vi "XUVCCDRotate.vi"() -> ()   [LabVIEW 2017]
uses:
  <vilib>/Utility/file.llb/Write Delimited Spreadsheet (DBL).vi
  atmcd32d.dll
panel:
  out "Array":dbl[](array[numeric])
  in  "Nb of steps":i32=50000
  out "Current position":dbl
  in  "Step size (deg.)":dbl=10.0
  out "Is Ready?":bool
  out "VISA resource name":refnum<visa-resource-name>="ASRL7::INSTR"
  out "Connected":bool
  in  "start":bool
  in  "?":bool
  out "Status":u32
  out "Get Status":u32
  out "Vertical Binned Waveform Graph":i32[](graph)
  in  "Numeric":dbl
  out "Intensity Graph":i32[][](graph)
  out "Set Image":u32
  out "Set Gate Mode":u32
  out "Shut Down":u32
  out "Detector Y Pixels":i32
  out "Get Detector":u32
  out "Set Exposure Time":u32
  out "Set Trigger Mode":u32
  out "Set Readout Mode":u32
  out "Set Acquisition Mode":u32
  out "Check Timings":u32
  out "Detector X Pixels":i32
  out "Start Acquisition":u32
  out "Get Acquired Data":u32
  out "Calculated Exposure Value":sgl format="%.5f"
  in  "Exposure Time (secs)":sgl format="%.2f"
  out "Initialize":u32
  in  "Trigger":u32(ring) items=["Internal", "External"]
  # "Status"
  # "Return values"
  # "USB iStarIMAG32at.VI"
  # "Acquisition Mode: Single Scan\nReadout Mode: Full Resolution Image"
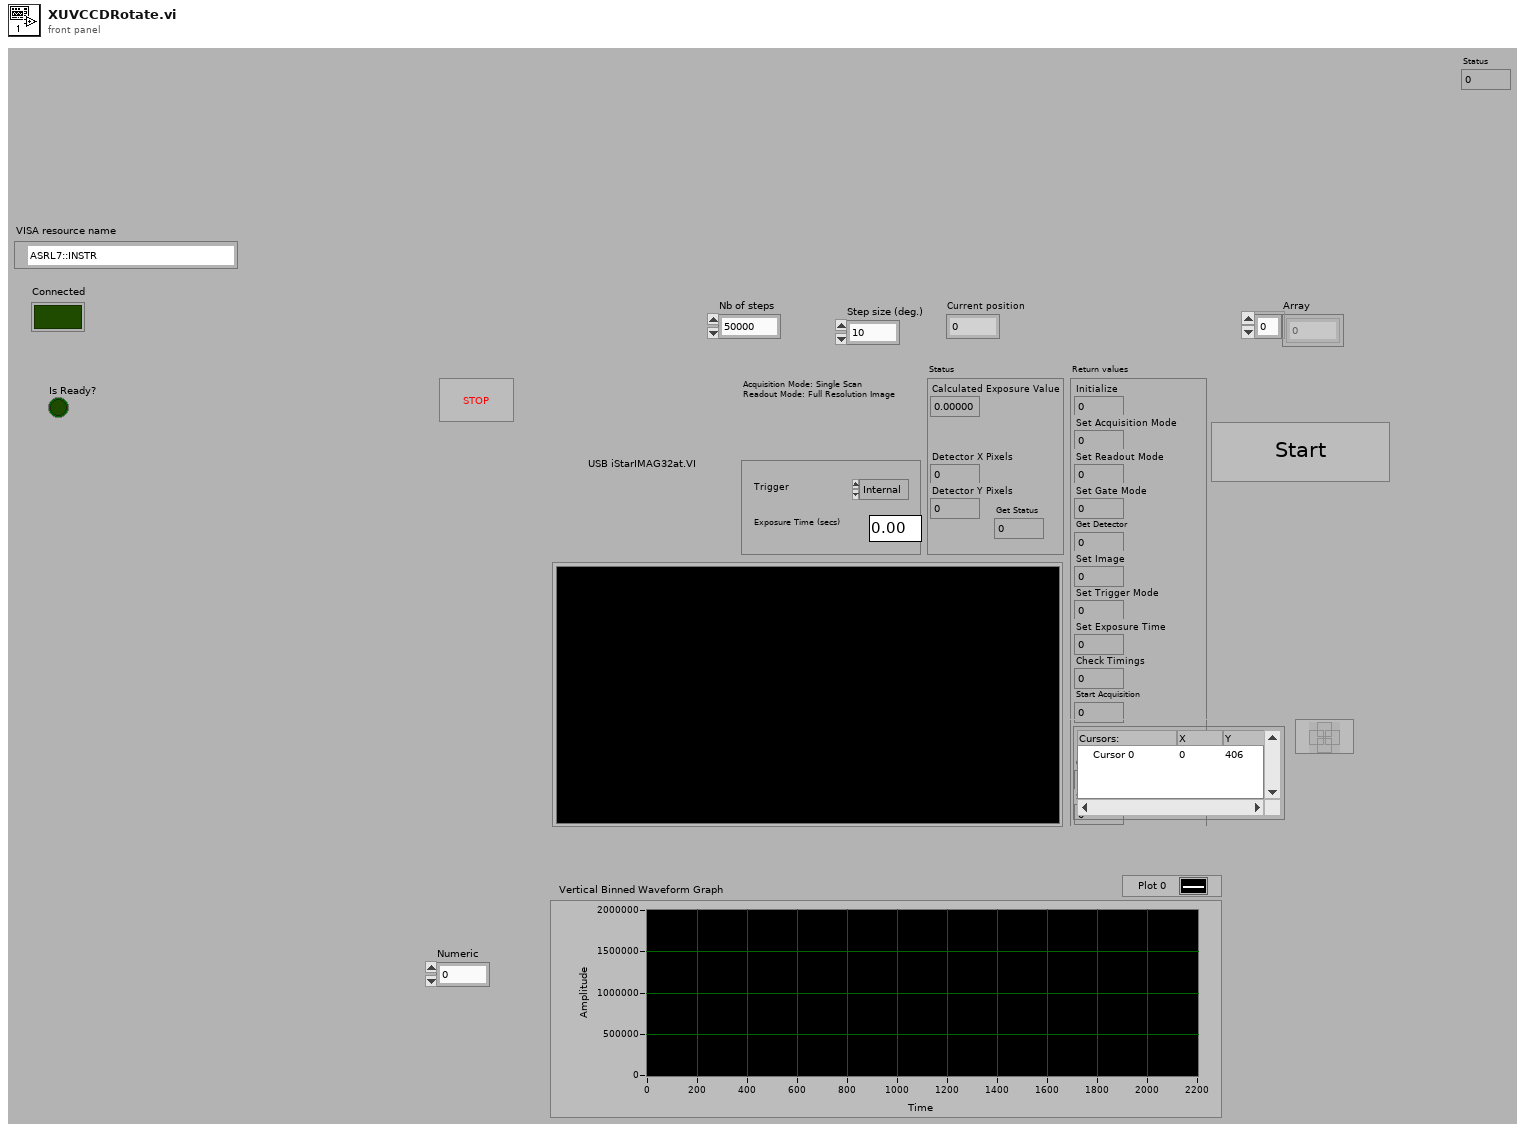
[diagram p1: front panel]
types:
  T1 = cluster{"VISA resource name":refnum<visa-resource-name>, "Device name":string, "Controller address":i32, "error":errorcluster}
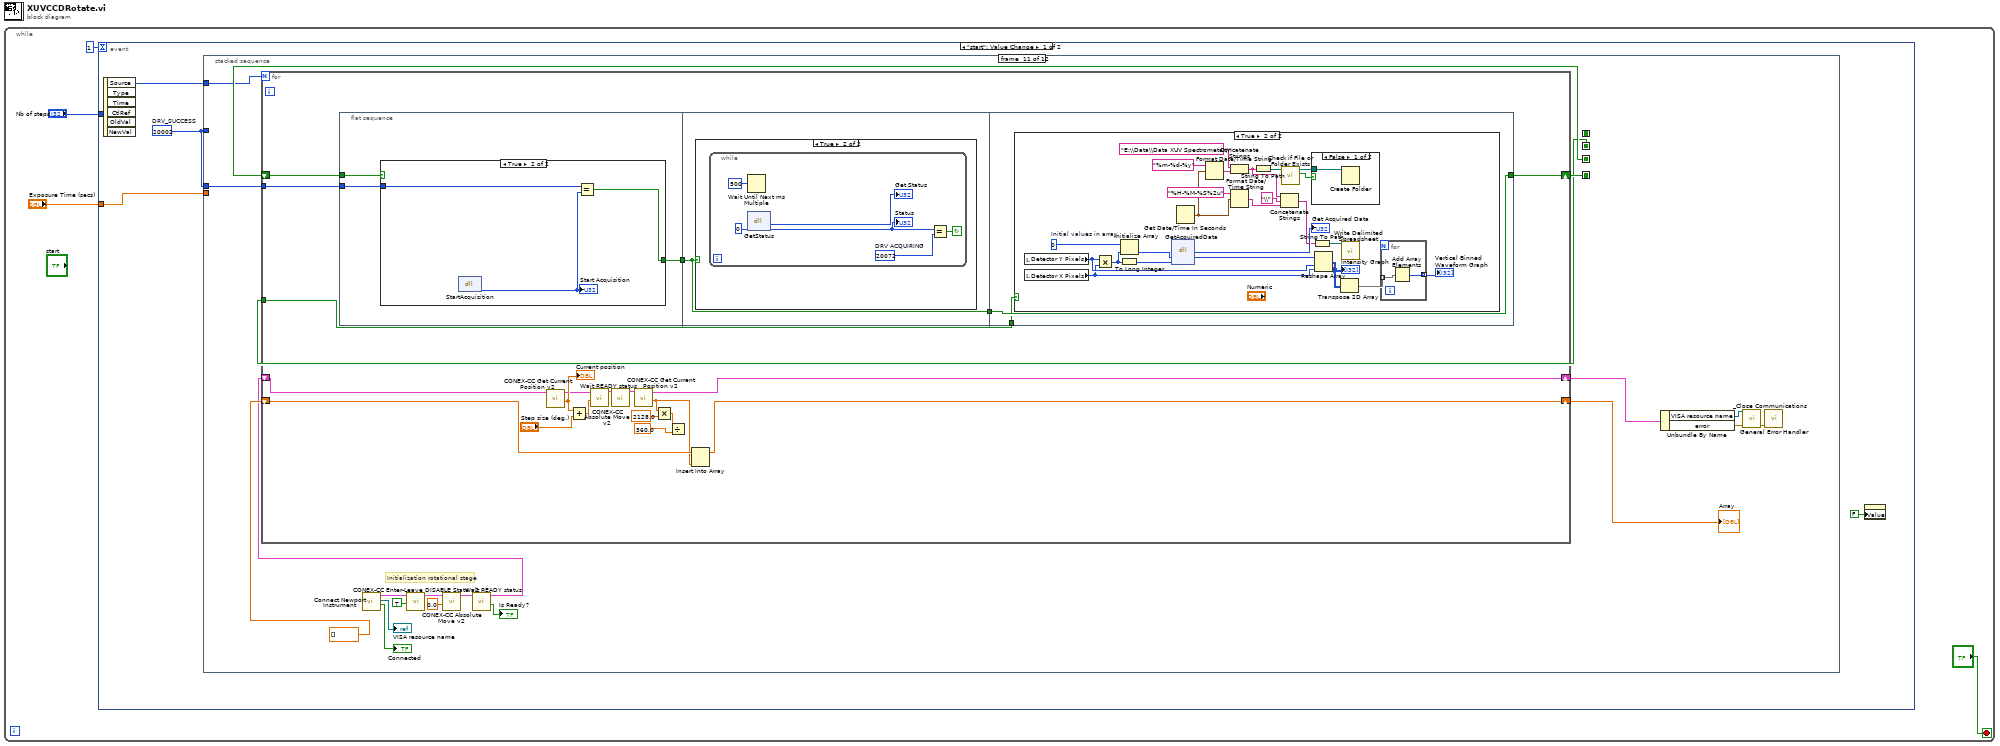
[diagram p0: block diagram]
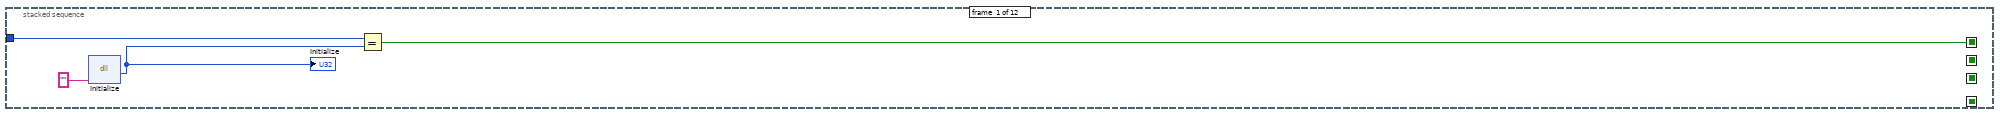
[diagram p2: hidden frame]
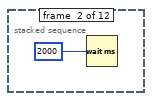
[diagram p3: hidden frame]
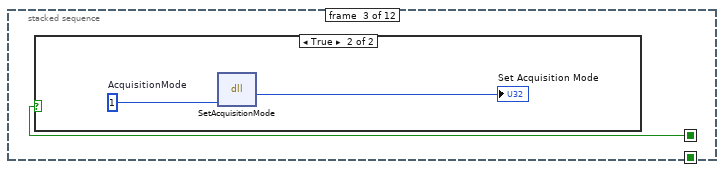
[diagram p4: hidden frame]
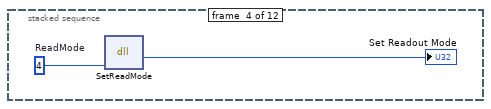
[diagram p6: hidden frame]
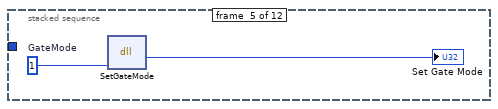
[diagram p7: hidden frame]
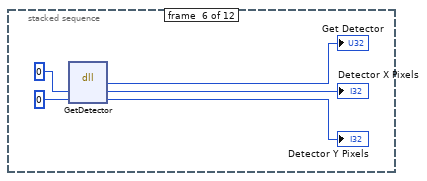
[diagram p8: hidden frame]
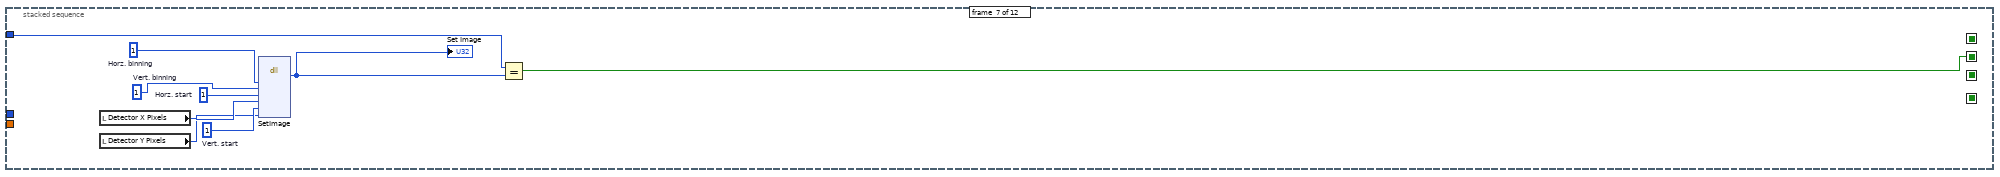
[diagram p9: hidden frame]
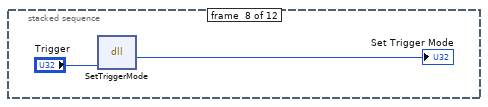
[diagram p10: hidden frame]
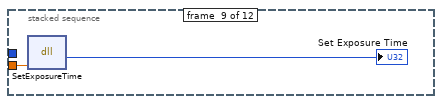
[diagram p11: hidden frame]
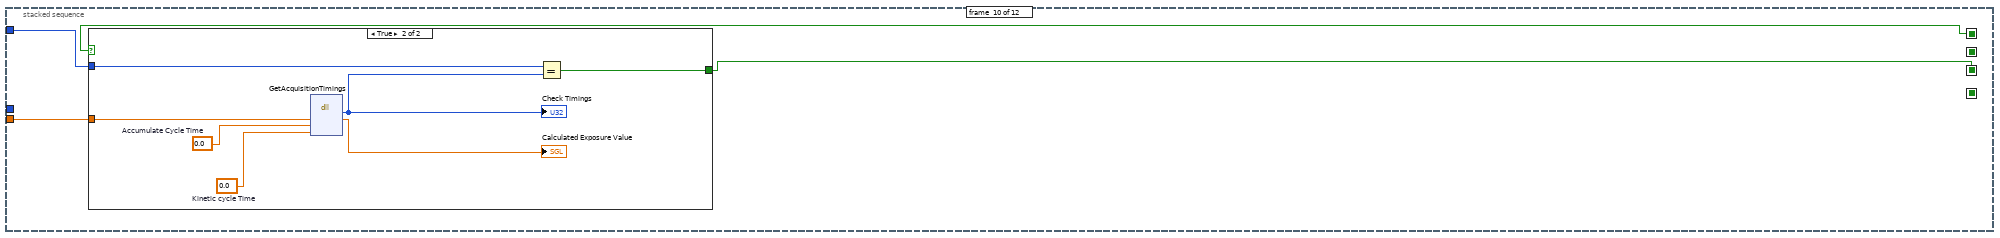
[diagram p12: hidden frame]
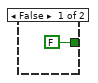
[diagram p13: hidden frame]
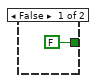
[diagram p14: hidden frame]
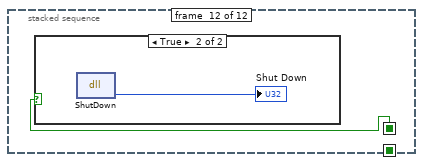
[diagram p18: hidden frame]
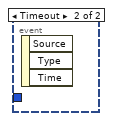
[diagram p20: hidden frame]
diagram:
  n1 = while {
    stop <- "?" stop-if-true
    n2 = event shown="[0] \"start\": Value Change" {
      selector: _ -> [_ _]
      dyn-events: _ -> [_ _]
      timeout: 1 -> [_ _]
      tunnel: "Exposure Time (secs)" -> [w8 _]
      tunnel: "Nb of steps" -> [w6 _]
      event "start": Value Change {
        w7 = 20002  # DRV_SUCCESS
        n3 = event-data() -> ()  [unwired: 1 in, 6 out]
        n4 = stacked-sequence {
          seq-local: [w10 _ _ _ _ _ _ _ _ _ _ _] -> [_ _ w14 _ _ _ _ _ _ w39 _ w134]
          seq-local: [_ _ _ _ _ _ _ _ _ w40 _ _] -> [_ _ _ _ _ _ _ _ _ _ w70 _]
          seq-local: [_ _ _ _ _ _ _ _ _ _ w68 _] -> [_ _ _ _ _ _ _ _ _ _ _ _]
          seq-local: [_ _ _ _ _ _ w26 _ _ _ _ _] -> [_ _ _ _ _ _ _ _ _ _ w67 _]
          tunnel: w8 -> [_ _ _ _ _ _ _ _ w38 w42 _ _]
          tunnel: w7 -> [w11 _ _ _ _ _ w28 _ _ w41 _ _]
          tunnel: w7 -> [_ _ _ _ _ _ _ _ _ _ w69 _]
          tunnel: w6 -> [_ _ _ _ _ _ _ _ _ _ w52 _]
          frame #0 {
            n5 = dll-call lib="atmcd32d.dll" fn="Initialize" label="Call Library Function Initialize"("") -> (w12:u32)  [unwired: 4 in, 2 out]
            "Initialize" <- w12
            n6 = Equal?(x=w11, y=w12) -> (x = y?=w10:bool)
          }
          frame #1 {
            n7 = Wait (ms)(milliseconds to wait=u32 2000) -> ()  [unwired: 1 out]
          }
          frame #2 {
            n8 = case shown="True" w14 {
              frame False {
              }
              frame True {
                w16 = u16 1  # AcquisitionMode
                n9 = dll-call lib="atmcd32d.dll" fn="SetAcquisitionMode" label="Call Library Function SetAcquisitionMode"(w16) -> (→"Set Acquisition Mode":u32)  [unwired: 4 in, 2 out]
              }
            }
          }
          frame #3 {
            w18 = u16 4  # ReadMode
            n10 = dll-call lib="atmcd32d.dll" fn="SetReadMode" label="Call Library Function SetReadMode"(w18) -> (→"Set Readout Mode":u32)  [unwired: 4 in, 2 out]
          }
          frame #4 {
            w20 = u16 1  # GateMode
            n11 = dll-call lib="atmcd32d.dll" fn="SetGateMode" label="Call Library Function SetGateMode"(w20) -> (→"Set Gate Mode":u32)  [unwired: 4 in, 2 out]
          }
          frame #5 {
            n12 = dll-call lib="atmcd32d.dll" fn="GetDetector" label="Call Library FunctionGetDetector"(i16 0, i16 0) -> (→"Get Detector":u32, →"Detector X Pixels":i32, →"Detector Y Pixels":i32)  [unwired: 3 in, 2 out]
          }
          frame #6 {
            w31 = u16 1  # Vert. start
            w32 = u16 1  # Horz. start
            w33 = u16 1  # Vert. binning
            w34 = u16 1  # Horz. binning
            n13 = local read "Detector X Pixels"() -> (w30:i32)
            n14 = local read "Detector Y Pixels"() -> (w29:i32)
            n15 = dll-call lib="atmcd32d.dll" fn="SetImage" label="Call Library Function SetImage"(w34, w33, w32, w30, w31, w29) -> (w27:u32)  [unwired: 9 in, 2 out]
            "Set Image" <- w27
            n16 = Equal?(x=w28, y=w27) -> (x = y?=w26:bool)
          }
          frame #7 {
            n17 = dll-call lib="atmcd32d.dll" fn="SetTriggerMode" label="Call Library Function SetTrigger Mode"("Trigger") -> (→"Set Trigger Mode":u32)  [unwired: 4 in, 2 out]
          }
          frame #8 {
            n18 = dll-call lib="atmcd32d.dll" fn="SetExposureTime" label="Call Library FunctionSet Exposure Time"(w38) -> (→"Set Exposure Time":u32)  [unwired: 4 in, 2 out]
          }
          frame #9 {
            n19 = case shown="True" w39 {
              tunnel: w42 -> [_ w47]
              tunnel: w41 -> [_ w44]
              tunnel: [FALSE w46] -> w40
              frame False {
              }
              frame True {
                w49 = sgl 0.0  # Accumulate Cycle Time
                w50 = sgl 0.0  # Kinetic cycle Time
                n20 = dll-call lib="atmcd32d.dll" fn="GetAcquisitionTimings" label="Call Library Function Check Timings"(w47, w49, w50) -> (w45:u32, →"Calculated Exposure Value":sgl)  [unwired: 5 in, 2 out]
                "Check Timings" <- w45
                n21 = Equal?(x=w44, y=w45) -> (x = y?=w46:bool)
              }
            }
          }
          frame #10 {
            # "Initialization rotational stage"
            n22 = call <userlib>:"Connect Newport Instrument.vi"() -> ("Connected"=→"Connected":bool, "VISA resource name (duplicate)"=→"VISA resource name":refnum<visa-resource-name>, "Device Connection Cluster"=w62:T1)  [unwired: 7 in, 2 out]
            n23 = call <userlib>:"CONEX-CC Enter-Leave DISABLE State v2.vi"("Ready? (false=DISABLE true=READY)"=TRUE, "Connection Cluster in"=w62) -> ("Connection Cluster out"=w63:T1)  [unwired: 7 in]
            n24 = call <userlib>:"CONEX-CC Absolute Move v2.vi"("Target position"=0.0, "Connection Cluster in"=w63) -> ("Connection Cluster out"=w64:T1)  [unwired: 7 in]
            n25 = call <userlib>:"Wait READY status.vi"("Connection Cluster in"=w64) -> ("IsReady?"=→"Is Ready?":bool, "Connection Cluster out"=w57:T1)  [unwired: 9 in]
            n26 = for {
              N: w52 -> [_]
              tunnel: w69 -> [w89]
              tunnel: w67 -> [w87]
              shift-right: [w88] -> w68
              shift-left: w70 -> [w90]
              shift-right: [w83] -> w51
              shift-left: dbl[] [] -> [w85]
              shift-right: [w84] -> w53
              shift-left: w57 -> [w86]
              n27 = flat-sequence {
                tunnel: w90 -> [w93]
                tunnel: w89 -> [w92]
                tunnel: [w91] -> w82
                tunnel: w82 -> [w98]
                tunnel: [w98] -> w81
                tunnel: [w106] -> w88
                tunnel: w81 -> [w106]
                tunnel: w87 -> [w105]
                frame #0 {
                  n28 = case shown="True" w93 {
                    tunnel: [FALSE w96] -> w91
                    tunnel: w92 -> [_ w95]
                    frame False {
                    }
                    frame True {
                      n29 = dll-call lib="atmcd32d.dll" fn="StartAcquisition" label="Call Library Function start acquisition"() -> (w97:u32)  [unwired: 3 in, 2 out]
                      "Start Acquisition" <- w97
                      n30 = Equal?(x=w95, y=w97) -> (x = y?=w96:bool)
                    }
                  }
                }
                frame #1 {
                  n31 = case shown="True" w98 {
                    frame False {
                    }
                    frame True {
                      n32 = while {
                        stop <- w102 continue-if-true
                        w101 = u16 20072  # DRV ACQUIRING
                        n33 = Wait Until Next ms Multiple(millisecond multiple=u32 500) -> ()  [unwired: 1 out]
                        n34 = dll-call lib="atmcd32d.dll" fn="GetStatus" label="Call Library Function GetAcquisitionStatus"(u16 0) -> (→"Get Status":u32, w100:u32)  [unwired: 3 in, 2 out]
                        "Status" <- w100
                        n35 = Equal?(x=w100, y=w101) -> (x = y?=w102:bool)
                      }
                    }
                  }
                }
                frame #2 {
                  n36 = case shown="True" w105 {
                    frame False {
                    }
                    frame True {
                      w130 = 0  # Initial values in array
                      n37 = local read "Detector Y Pixels"() -> (w124:i32)
                      n38 = local read "Detector X Pixels"() -> (w123:i32)
                      n39 = Multiply(x=w124, y=w123) -> (x*y=w126:i32)
                      n40 = To Long Integer(number=w126) -> (32bit integer=w127:i32)
                      n41 = Initialize Array "Initialize Array"(w130, w126) -> (w128:i32[])
                      n42 = dll-call lib="atmcd32d.dll" fn="GetAcquiredData" label="Call Library Function Get Acquired data"(w128, w127) -> (→"Get Acquired Data":u32, w125:i32[])  [unwired: 4 in, 2 out]
                      n43 = Get Date/Time In Seconds() -> (seconds since 1Jan1904=w120:timestamp)
                      n44 = Format Date/Time String(time format string (%c)="%m-%d-%y", seconds (now)=w120) -> (date/time string=w118:string)  [unwired: 1 in]
                      n45 = Concatenate Strings("E:\\Data\\Data XUV Spectrometer\\" ("string"), w118) -> (w121:string)
                      n46 = Format Date/Time String(time format string (%c)="%H-%M-%S%2u", seconds (now)=w120) -> (date/time string=w119:string)  [unwired: 1 in]
                      n47 = String To Path(string=w121) -> (path=w117:path)
                      n48 = Concatenate Strings(w121, "\\" ("string"), w119) -> (w122:string)
                      n49 = call <vilib>:"Check if File or Folder Exists.vi"("path"=w117) -> ("file or folder exists?"=w115:bool, "dup path"=w116:path)  [unwired: 8 in, 1 out]
                      n50 = case shown="False" w115 {
                        tunnel: w116 -> [w133 _]
                        frame False {
                          n51 = Create Folder(path (use dialog)=w133) -> ()  [unwired: 2 in, 3 out]
                        }
                        frame True {
                        }
                      }
                      n52 = String To Path(string=w122) -> (path=w110:path)
                      n53 = Reshape Array(w125, w124, w123) -> (w109:i32[][])
                      "Intensity Graph" <- w109
                      n54 = Transpose 2D Array(2D array=w109) -> (transposed array=w107:i32[][])
                      n55 = call-poly <vilib>:"Write Delimited Spreadsheet.vi"("file path (dialog if empty)"=w110) -> ()  [unwired: 13 in, 2 out]
                      n56 = for {
                        tunnel: w107 -> [w132] mode=indexing
                        tunnel: [w131] -> w108 mode=indexing
                        n57 = Add Array Elements(numeric array=w132) -> (sum=w131:i32)
                      }
                      "Vertical Binned Waveform Graph" <- w108
                    }
                  }
                }
              }
              n58 = call <userlib>:"CONEX-CC Get Current Position v2.vi"("Connection Cluster in"=w86) -> ("Current position"=w76:dbl, "Connection Cluster out"=w75:T1)  [unwired: 8 in, 1 out]
              "Current position" <- w76
              n59 = Add(x=w76, y="Step size (deg.)") -> (x+y=w78:dbl)
              n60 = call <userlib>:"CONEX-CC Absolute Move v2.vi"("Target position"=w78, "Connection Cluster in"=w75) -> ("Connection Cluster out"=w74:T1)  [unwired: 7 in]
              n61 = call <userlib>:"Wait READY status.vi"("Connection Cluster in"=w74) -> ("Connection Cluster out"=w79:T1)  [unwired: 9 in, 1 out]
              n62 = call <userlib>:"CONEX-CC Get Current Position v2.vi"("Connection Cluster in"=w79) -> ("Current position"=w71:dbl, "Connection Cluster out"=w84:T1)  [unwired: 8 in, 1 out]
              n63 = Multiply(x=w71, y=2128.0) -> (x*y=w80:dbl)
              n64 = Divide(x=w80, y=360.0) -> ()  [unwired: 1 out]
              n65 = Insert Into Array(array=w85, new element=w71) -> (w83:dbl[])  [unwired: 1 in]
            }
            "Array" <- w51
            n66 = Unbundle By Name(w53) -> ("VISA resource name"=w54:refnum<visa-resource-name>, "error"=w55:errorcluster)
            n67 = call <userlib>:"_Close Communications.vi"("Instrument Channel"=w54, "error in (no error)"=w55) -> ("error out"=w56:errorcluster)  [unwired: 13 in]
            n68 = call <vilib>:"General Error Handler.vi"("error in (no error)"=w56) -> ()  [unwired: 10 in, 5 out]
          }
          frame #11 {
            n69 = case shown="True" w134 {
              frame False {
              }
              frame True {
                n70 = dll-call lib="atmcd32d.dll" fn="ShutDown" label="Call Library Function Shutdown"() -> (→"Shut Down":u32)  [unwired: 3 in, 2 out]
              }
            }
          }
        }
        n71 = property on="start" class="Bool (strict)"("Value"=FALSE ("Take image")) -> ()  [unwired: 2 in, 2 out]
      }
      event Timeout {
        n72 = event-data() -> ()  [unwired: 1 in, 3 out]
      }
    }
  }
